vi "Launch Are you Sure Dialog.vi"(4 "Error In":errorcluster) -> (0 "Error Out":errorcluster)   [LabVIEW 2014, in "Dialog Boxes.lvlib"]
uses:
  Dialog Boxes.lvlib
  _dialogs/Simple Quit Verification.vi
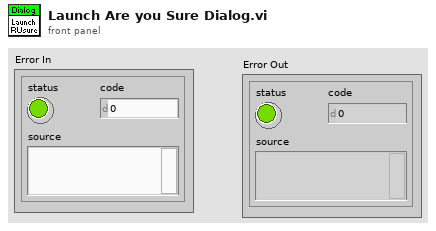
[diagram p1: front panel]
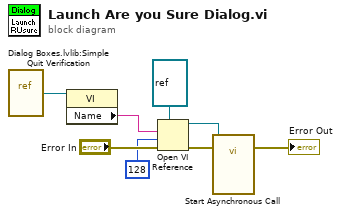
[diagram p0: block diagram]
diagram:
  n1 = vi-ref "Dialog Boxes.lvlib:Simple Quit Verification.vi"() -> (w8:refnum<vi>)
  n2 = property class="VI"(reference=w8) -> ("Name"=w7:string)  [unwired: 1 in, 2 out]
  n3 = Open VI Reference(type specifier VI Refnum (for type only)=refnum<vi> refnum, vi path=w7, options=128, error in (no error)="Error In") -> (vi reference=w4:refnum<vi>, error out=w5:errorcluster)  [unwired: 2 in]
  n4 = call-by-ref "Start Asynchronous Call"(reference=w4, error in=w5) -> (error out=→"Error Out":errorcluster)  [unwired: 12 in, 1 out]
